vi "VCS Get Version.vi"(8 "error in (no error)":errorcluster, 11 "axis In":cluster{"keyHandle":u32, "nodeId":u16}={"keyHandle"=0, "nodeId"=1}) -> (0 "error out":errorcluster, 2 "version numbers":T1 {"applicationVersion" format="%x"; "applicationNumber" format="%x"; "softwareVersion" format="%x"; "hardwareVersion" format="%x"}, 3 "axis Out":cluster{"keyHandle":u32, "nodeId":u16}={"keyHandle"=0, "nodeId"=1})   [LabVIEW 2018]
doc: "<B>VCS GetVersion</B> returns the firmware version."
uses:
  Resources/EposCmd.dll
  Resources/EposCmd64.dll
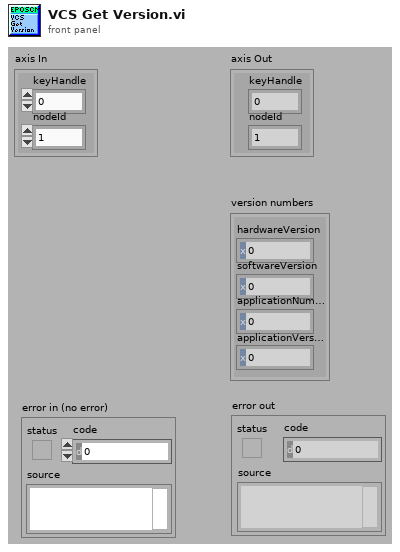
[diagram p1: front panel]
types:
  T1 = cluster{"hardwareVersion ":u16, "softwareVersion ":u16, "applicationNumber":u16, "applicationVersion":u16}
  T2 = cluster{"pHardwareVersion":u16, "pSoftwareVersion":u16, "pApplicationNumber":u16, "pApplicationVersion":u16}
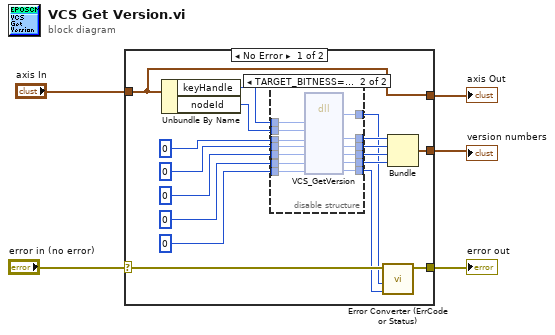
[diagram p0: block diagram]
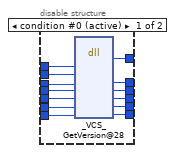
[diagram p2: hidden frame]
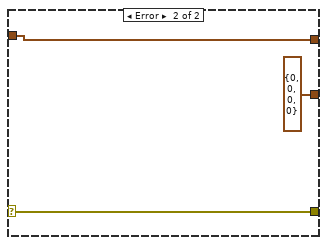
[diagram p3: hidden frame]
diagram:
  n1 = case shown="No Error" "error in (no error)" {
    selector: "error in (no error)" -> [w22 w51]
    tunnel: [w21 w51] -> w4
    tunnel: "axis In" -> [w7 w50]
    tunnel: [w8 T2 {"pHardwareVersion"=0, "pSoftwareVersion"=0, "pApplicationNumber"=0, "pApplicationVersion"=0}] -> w2
    tunnel: [w7 w50] -> w1
    frame No Error {
      n2 = Unbundle By Name(w7) -> ("keyHandle"=w18:u32, "nodeId"=w17:u16)
      n3 = disable-structure shown="TARGET_BITNESS==64" {
        disable-tunnel: [w35 w48] -> w20
        disable-tunnel: u32 0 ("pErrorCode") -> [w34 w47]
        disable-tunnel: w18 -> [w33 w46]
        disable-tunnel: w17 -> [w32 w45]
        disable-tunnel: u16 0 ("hardware Version") -> [w31 w44]
        disable-tunnel: u16 0 ("software Version") -> [w30 w43]
        disable-tunnel: u16 0 ("application number") -> [w29 w42]
        disable-tunnel: u16 0 ("application version") -> [w28 w41]
        disable-tunnel: [w27 w40] -> w12
        disable-tunnel: [w26 w39] -> w11
        disable-tunnel: [w25 w38] -> w10
        disable-tunnel: [w24 w37] -> w9
        disable-tunnel: [w23 w36] -> w6
        frame condition #0 (active) {
          n4 = dll-call lib="C:/Projeto em LabVIEW/EPOS-LabVIEW-Instrument-Driver-En/LabVIEW/maxon EPOS/Resources/EposCmd.*" fn="_VCS_GetVersion@28"("KeyHandle"=w33, "NodeId"=w32, "pHardwareVersion"=w31, "pSoftwareVersion"=w30, "pApplicationNumber"=w29, "pApplicationVersion"=w28, "pErrorCode"=w34) -> (w23:i32, "pHardwareVersion"=w27:u16, "pSoftwareVersion"=w26:u16, "pApplicationNumber"=w25:u16, "pApplicationVersion"=w24:u16, "pErrorCode"=w35:u32)  [unwired: 5 in, 2 out]
        }
        frame condition #1 {
          n5 = dll-call lib="C:/setup/Resources/EposCmd64.*" fn="VCS_GetVersion" ("EposCmd.dll:_VCS_GetVersion@28")("KeyHandle"=w46, "NodeId"=w45, "pHardwareVersion"=w44, "pSoftwareVersion"=w43, "pApplicationNumber"=w42, "pApplicationVersion"=w41, "pErrorCode"=w47) -> ("Rückgabetyp"=w36:i32, "pHardwareVersion"=w40:u16, "pSoftwareVersion"=w39:u16, "pApplicationNumber"=w38:u16, "pApplicationVersion"=w37:u16, "pErrorCode"=w48:u32)  [unwired: 5 in, 2 out]
        }
      }
      n6 = call "Error Converter (ErrCode or Status).vi"("error code"=w20, "return type"=w6, "error in (no error)"=w22) -> ("error out"=w21:errorcluster)  [unwired: 7 in]
      n7 = Bundle("pHardwareVersion"=w12, "pSoftwareVersion"=w11, "pApplicationNumber"=w10, "pApplicationVersion"=w9) -> (w8:T2)  [unwired: 1 in]
    }
    frame Error {
    }
  }
  "error out" <- w4
  "axis Out" <- w1
  "version numbers" <- w2
